vi "Parse Test Mode.vi"(8 "error in (no error)":errorcluster, 11 "SPECAN_PVT in":refnum<class "SPECAN_PVT.lvclass">) -> (0 "error out":errorcluster, 3 "SPECAN_PVT out":refnum<class "SPECAN_PVT.lvclass">)   [LabVIEW 2018, in "SPECAN_PVT.lvlib" / "SPECAN_PVT.lvclass"]
uses:
  SPECAN_PVT.lvclass
  C:/Sequence Automation/Plugins/Measurement Interface.lvlibp/Measurement Interface.lvclass
  SPECAN_PVT.lvclass/SPECAN_PVT.ctl
  Plugins/Measurement Interface.lvlibp/Private Methods/Measurement Name/Read Measurement Name.vi
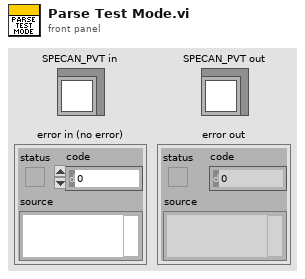
[diagram p1: front panel]
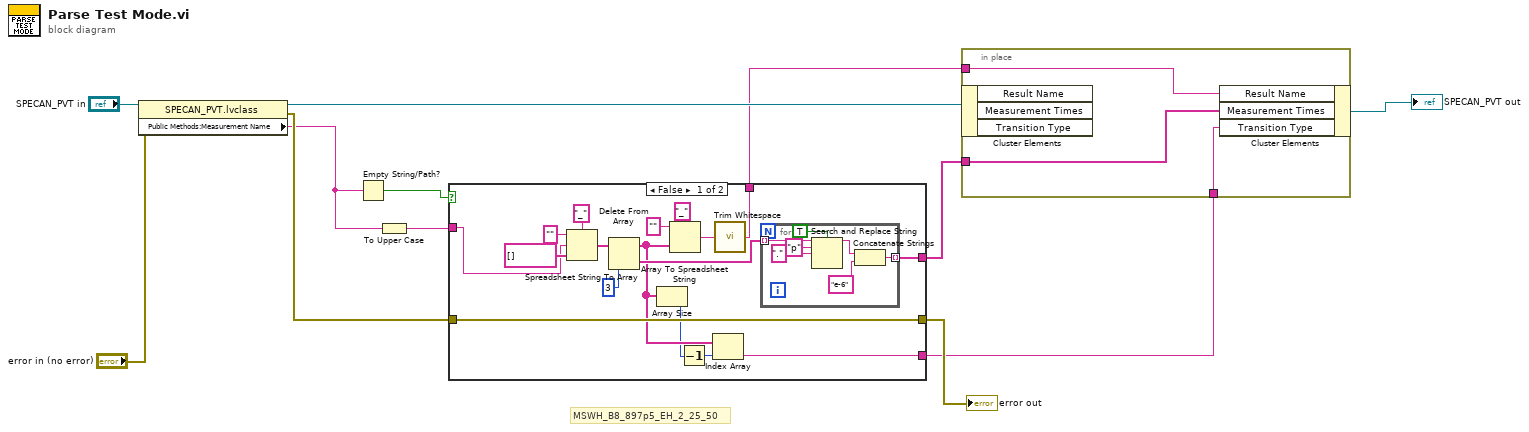
[diagram p0: block diagram]
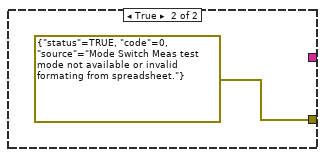
[diagram p2: hidden frame]
diagram:
  # "MSWH_B8_897p5_EH_2_25_50"
  n1 = property class="SPECAN_PVT.lvclass"(reference="SPECAN_PVT in", error in="error in (no error)") -> (reference out=w8:refnum<class "SPECAN_PVT.lvclass">, error out=w12:errorcluster, "Public Methods:Measurement Name"=w3:string)
  n2 = Empty String/Path?(string/path=w3) -> (empty?=w2:bool)
  n3 = To Upper Case(1:w3) -> (0:w5:string)
  n4 = case shown="False" w2 {
    tunnel: w12 -> [w29 _]
    tunnel: [w29 errorcluster {"status"=TRUE, "code"=0, "source"="Mode Switch Meas test mode not available or invalid formating from spreadsheet."} ("error out")] -> w10
    tunnel: w5 -> [w22 _]
    tunnel: [w23 _] -> w6
    tunnel: [w17 _] -> w4
    tunnel: [w13 _] -> w1
    frame False {
      n5 = Spreadsheet String To Array(delimiter (Tab)="_", format string="", spreadsheet string=w22, array type (2D Dbl)=string[] []) -> (array=w25:string[])
      n6 = Delete From Array(array=w25, length=3) -> (deleted portion=w24:string[], array with subset deleted=w16:string[])  [unwired: 1 in]
      n7 = Array Size(array=w16) -> (size(s)=w15:i32)
      n8 = Array To Spreadsheet String(delimiter (Tab)="_", array=w16, 3:"" ("format string")) -> (spreadsheet string=w19:string)
      n9 = Decrement(x=w15) -> (x-1=w14:i32)
      n10 = Index Array(array=w16, index=w14) -> (element=w13:string)
      n11 = call <vilib>:"Trim Whitespace.vi"("string"=w19) -> ("trimmed string"=w17:string)  [unwired: 1 in]
      n12 = for {
        tunnel: w24 -> [w33] mode=indexing
        tunnel: [w35] -> w23 mode=indexing
        n13 = Search and Replace String(case sensitive?=TRUE ("ignore case? (F)"), input string=w33, search string="p", replace string="." ("replace string (\"\")")) -> (result string=w34:string)  [unwired: 4 in, 3 out]
        n14 = Concatenate Strings(w34, "e-6" ("string")) -> (w35:string)
      }
    }
    frame True {
    }
  }
  "error out" <- w10
  n15 = in-place {
    in-place-border: w4 -> [w40]
    in-place-border: w6 -> [w39]
    in-place-border: w1 -> [w38]
    n16 = in-place-cluster #1(w8) -> ()  [unwired: 3 out]
    n17 = in-place-cluster #1("Result Name"=w40, "Measurement Times"=w39, "Transition Type"=w38) -> (→"SPECAN_PVT out":refnum<class "SPECAN_PVT.lvclass">)
  }
